vi "대회용.vi"() -> ()   [LabVIEW 2015]
uses:
  <vilib>/NXT/Block Support/NXT_OutputPort.ctl
  <vilib>/NXT/Block Support/NXT_InputPort.ctl
  <vilib>/NXT/Dual Mode Library/Sensors/EV3_Ultrasonic_CM.vi
  <vilib>/NXT/NXTIO Xnodes/NXTIONodeSubVIs/NXTMoveMotors.vi
  <vilib>/NXT/Dual Mode Library/Waits/Wait_Num.vi
  <vilib>/NXT/Dual Mode Library/Sensors/EV3_Color_Reflect.vi
  <vilib>/NXT/Subs/LVHSConnector.ctl
  <vilib>/NXT/NXTIO Xnodes/NXTIOXNode/NXTIO.xnode
  <vilib>/NXT/LegoClasses/BrickReference/BrickReference.lvclass
panel:
  in  "Power/Speed 20":i8=75
  in  "Motors 10":T1=2 items=["Port A", "Port B", "Port C", "Port D"]
  in  "Time (1 sec) 10":sgl=1.0
  in  "Power/Speed 19":i8=75
  in  "Power/Speed 18":i8=75
  in  "Motors 9":T1=2 items=["Port A", "Port B", "Port C", "Port D"]
  in  "Time (1 sec) 9":sgl=1.0
  in  "Power/Speed 17":i8=75
  in  "Power/Speed 16":i8=75
  in  "Motors 8":T1=2 items=["Port A", "Port B", "Port C", "Port D"]
  in  "Time (1 sec) 8":sgl=1.0
  in  "Power/Speed 15":i8=75
  in  "Power/Speed 14":i8=75
  in  "Motors 7":T1=2 items=["Port A", "Port B", "Port C", "Port D"]
  in  "Time (1 sec) 7":sgl=1.0
  in  "Power/Speed 13":i8=75
  in  "stop":bool
  in  "Power/Speed 1":i8=75
  in  "Motors":T1=2 items=["Port A", "Port B", "Port C", "Port D"]
  in  "Time (1 sec)":sgl=1.0
  in  "Power/Speed 6":i8=75
  in  "Power/Speed 2":i8=75
  in  "Motors 2":T1=2 items=["Port A", "Port B", "Port C", "Port D"]
  in  "Time (1 sec) 2":sgl=1.0
  in  "Power/Speed 7":i8=75
  in  "Power/Speed 3":i8=75
  in  "Motors 3":T1=2 items=["Port A", "Port B", "Port C", "Port D"]
  in  "Time (1 sec) 3":sgl=1.0
  in  "Power/Speed 8":i8=75
  in  "Power/Speed 4":i8=75
  in  "Motors 4":T1=2 items=["Port A", "Port B", "Port C", "Port D"]
  in  "Time (1 sec) 4":sgl=1.0
  in  "Power/Speed 9":i8=75
  in  "Power/Speed 5":i8=75
  in  "Motors 5":T1=2 items=["Port A", "Port B", "Port C", "Port D"]
  in  "Time (1 sec) 5":sgl=1.0
  in  "Power/Speed 10":i8=75
  in  "Power/Speed 11":i8=75
  in  "Motors 6":T1=2 items=["Port A", "Port B", "Port C", "Port D"]
  in  "Time (1 sec) 6":sgl=1.0
  in  "Power/Speed 12":i8=75
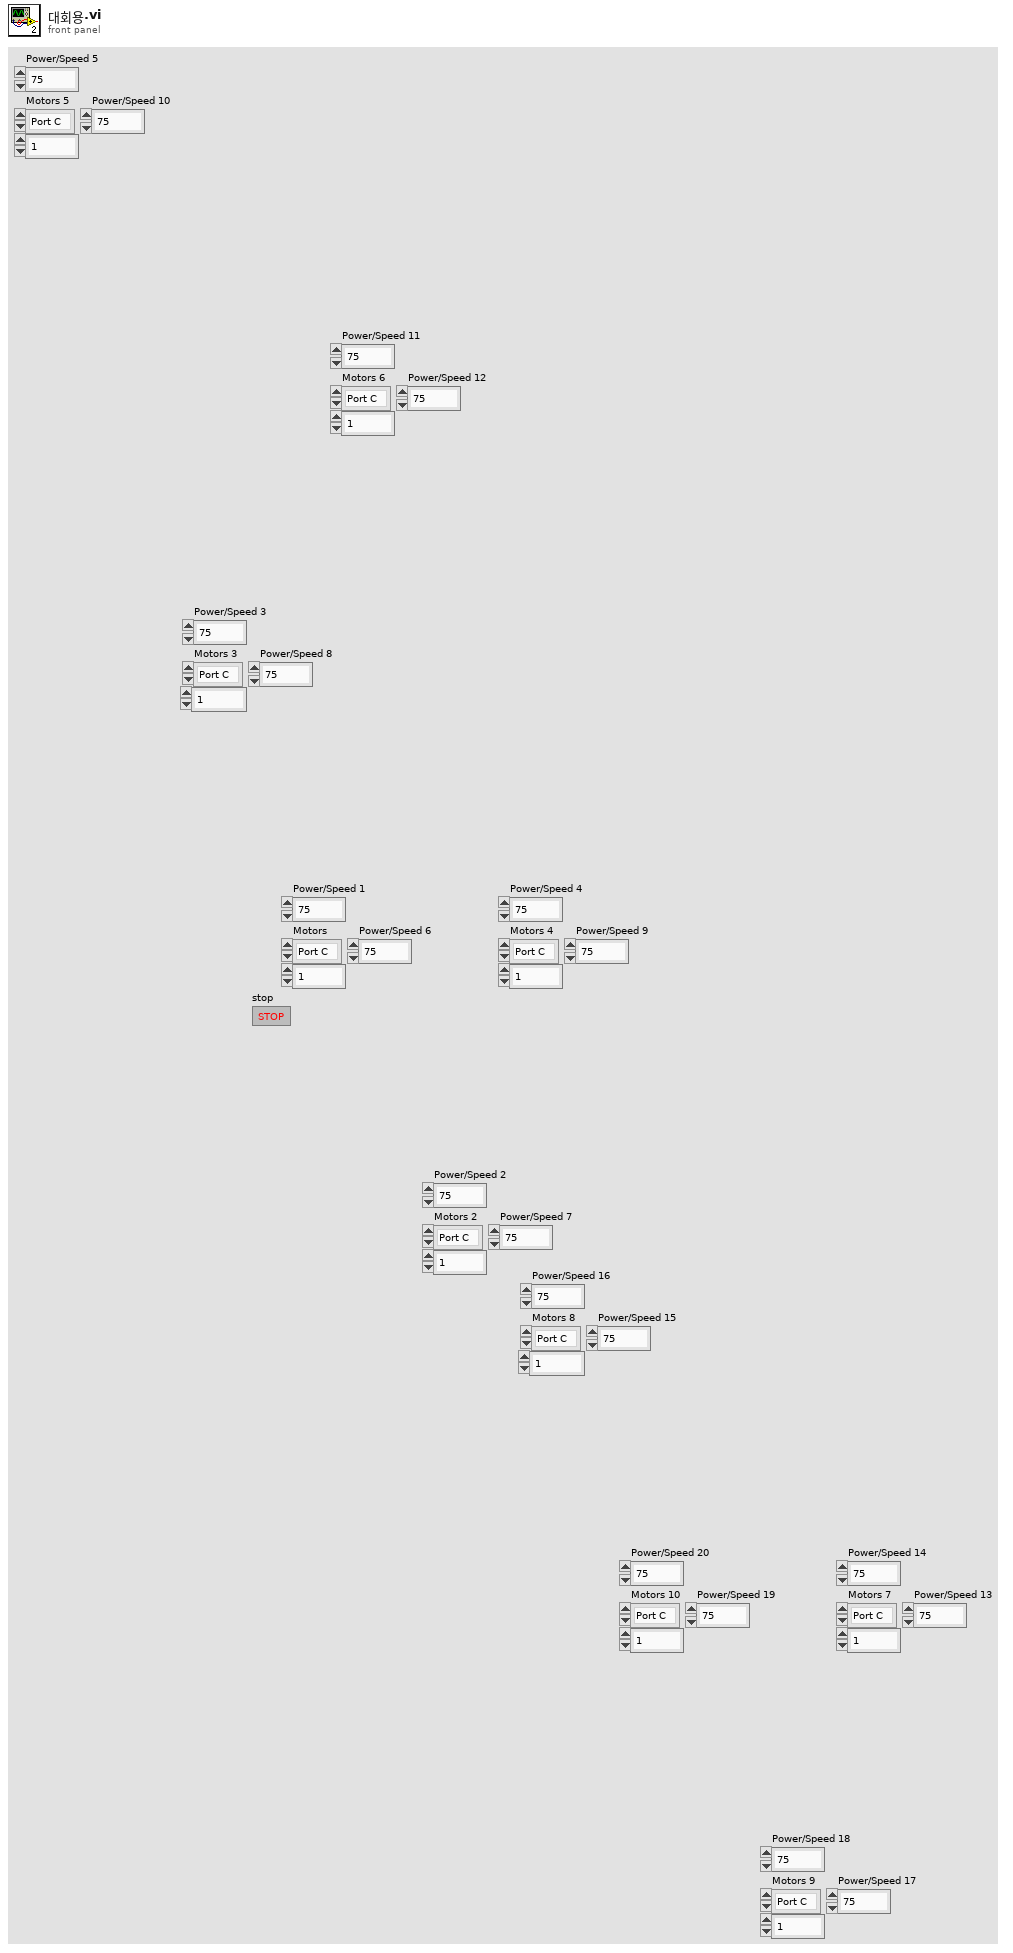
[diagram p1: front panel]
types:
  T1 = typedef "NXT_OutputPort.ctl" = u8
  T2 = typedef "NXT_InputPort.ctl" = u32
  T3 = typedef "LVHSConnector.ctl" = refnum<class "BrickReference.lvclass">
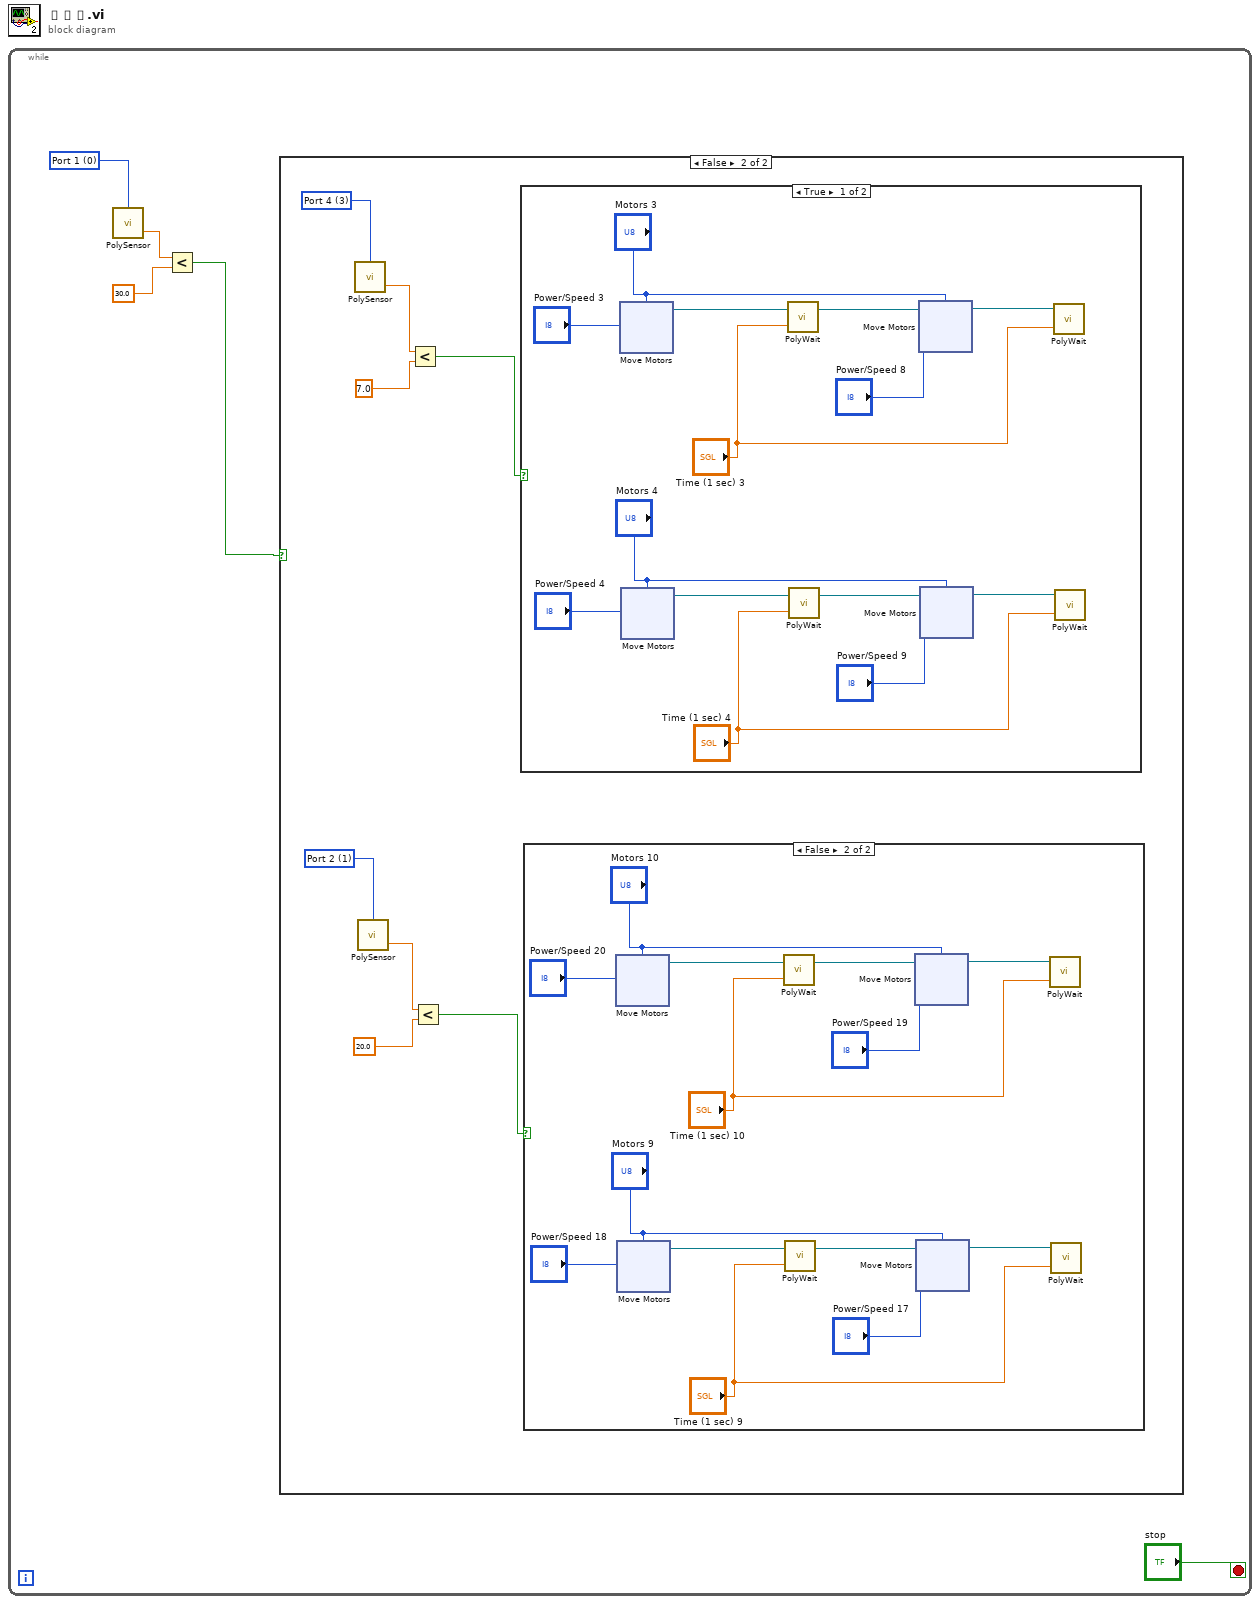
[diagram p0: block diagram]
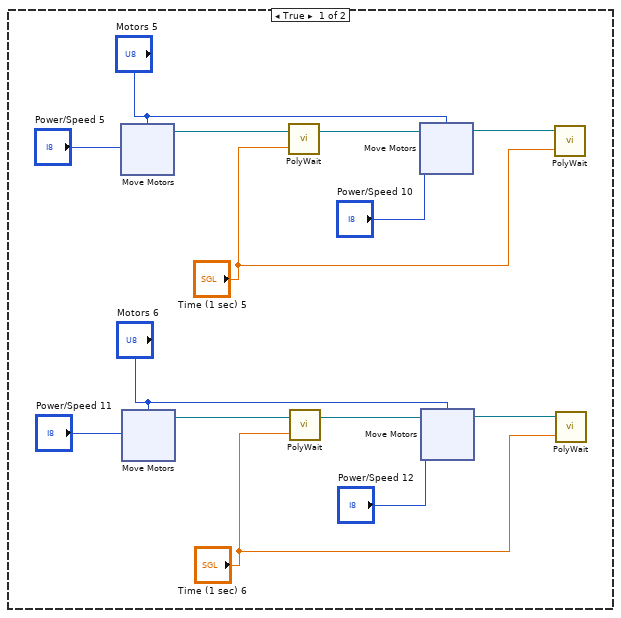
[diagram p2: hidden frame]
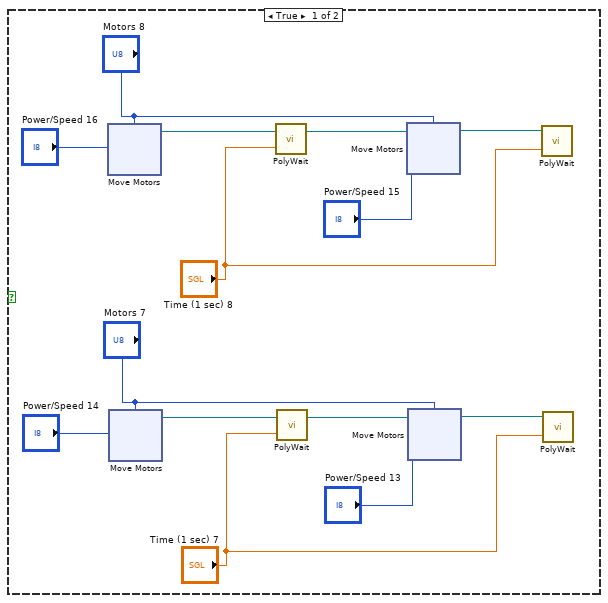
[diagram p3: hidden frame]
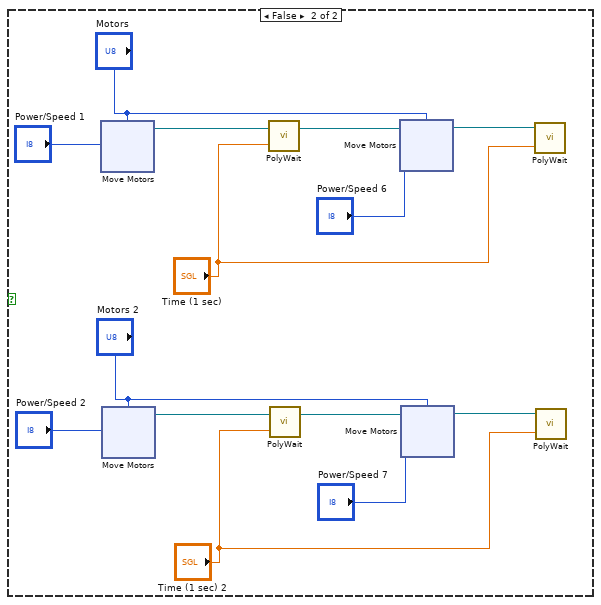
[diagram p4: hidden frame]
diagram:
  n1 = while {
    stop <- "stop" stop-if-true
    w2 = T2 0 items=["Port 1", "Port 2", "Port 3", "Port 4"] ("Port (Port 4)")
    n2 = call-poly <vilib>:"PolySensor.vi"("Port (Port 1)"=w2) -> ("Centimeters"=w4:sgl)  [unwired: 2 in, 1 out]
    n3 = Less?(x=w4, y=sgl 30.0) -> (x < y?=w1:bool)
    n4 = case shown="False" w1 {
      frame True {
        n5 = xnode "Move Motors"("Power/Speed 1"="Power/Speed 5", "Motors"="Motors 5") -> ("NXT/EV3"=w7:T3)  [unwired: 1 in]
        n6 = xnode "Move Motors"("Power/Speed 1"="Power/Speed 11", "Motors"="Motors 6") -> ("NXT/EV3"=w14:T3)  [unwired: 1 in]
        n7 = call-poly <vilib>:"PolyWait.vi"("Time (1 sec)"="Time (1 sec) 5", "NXT/EV3"=w7) -> ("NXT/EV3"=w11:T3)  [unwired: 2 in]
        n8 = call-poly <vilib>:"PolyWait.vi"("Time (1 sec)"="Time (1 sec) 6", "NXT/EV3"=w14) -> ("NXT/EV3"=w18:T3)  [unwired: 2 in]
        n9 = xnode "Move Motors"("Power/Speed 1"="Power/Speed 10", "Motors"="Motors 5", "NXT/EV3"=w11) -> ("NXT/EV3"=w10:T3)
        n10 = xnode "Move Motors"("Power/Speed 1"="Power/Speed 12", "Motors"="Motors 6", "NXT/EV3"=w18) -> ("NXT/EV3"=w17:T3)
        n11 = call-poly <vilib>:"PolyWait.vi"("Time (1 sec)"="Time (1 sec) 5", "NXT/EV3"=w10) -> ()  [unwired: 2 in, 1 out]
        n12 = call-poly <vilib>:"PolyWait.vi"("Time (1 sec)"="Time (1 sec) 6", "NXT/EV3"=w17) -> ()  [unwired: 2 in, 1 out]
      }
      frame False {
        w51 = T2 1 items=["Port 1", "Port 2", "Port 3", "Port 4"] ("Port (Port 4)")
        w55 = T2 3 items=["Port 1", "Port 2", "Port 3", "Port 4"] ("Port (Port 4)")
        n13 = call-poly <vilib>:"PolySensor.vi"("Port (Port 1)"=w55) -> ("Scaled Value"=w53:sgl)  [unwired: 2 in, 1 out]
        n14 = call-poly <vilib>:"PolySensor.vi"("Port (Port 1)"=w51) -> ("Scaled Value"=w49:sgl)  [unwired: 2 in, 1 out]
        n15 = Less?(x=w53, y=sgl 7.0) -> (x < y?=w52:bool)
        n16 = Less?(x=w49, y=sgl 20.0) -> (x < y?=w48:bool)
        n17 = case shown="True" w52 {
          frame True {
            n18 = xnode "Move Motors"("Power/Speed 1"="Power/Speed 3", "Motors"="Motors 3") -> ("NXT/EV3"=w152:T3)  [unwired: 1 in]
            n19 = xnode "Move Motors"("Power/Speed 1"="Power/Speed 4", "Motors"="Motors 4") -> ("NXT/EV3"=w145:T3)  [unwired: 1 in]
            n20 = call-poly <vilib>:"PolyWait.vi"("Time (1 sec)"="Time (1 sec) 3", "NXT/EV3"=w152) -> ("NXT/EV3"=w148:T3)  [unwired: 2 in]
            n21 = call-poly <vilib>:"PolyWait.vi"("Time (1 sec)"="Time (1 sec) 4", "NXT/EV3"=w145) -> ("NXT/EV3"=w141:T3)  [unwired: 2 in]
            n22 = xnode "Move Motors"("Power/Speed 1"="Power/Speed 8", "Motors"="Motors 3", "NXT/EV3"=w148) -> ("NXT/EV3"=w149:T3)
            n23 = xnode "Move Motors"("Power/Speed 1"="Power/Speed 9", "Motors"="Motors 4", "NXT/EV3"=w141) -> ("NXT/EV3"=w142:T3)
            n24 = call-poly <vilib>:"PolyWait.vi"("Time (1 sec)"="Time (1 sec) 3", "NXT/EV3"=w149) -> ()  [unwired: 2 in, 1 out]
            n25 = call-poly <vilib>:"PolyWait.vi"("Time (1 sec)"="Time (1 sec) 4", "NXT/EV3"=w142) -> ()  [unwired: 2 in, 1 out]
          }
          frame False {
            n26 = xnode "Move Motors"("Power/Speed 1"="Power/Speed 1", "Motors"="Motors") -> ("NXT/EV3"=w194:T3)  [unwired: 1 in]
            n27 = xnode "Move Motors"("Power/Speed 1"="Power/Speed 2", "Motors"="Motors 2") -> ("NXT/EV3"=w187:T3)  [unwired: 1 in]
            n28 = call-poly <vilib>:"PolyWait.vi"("Time (1 sec)"="Time (1 sec)", "NXT/EV3"=w194) -> ("NXT/EV3"=w190:T3)  [unwired: 2 in]
            n29 = call-poly <vilib>:"PolyWait.vi"("Time (1 sec)"="Time (1 sec) 2", "NXT/EV3"=w187) -> ("NXT/EV3"=w183:T3)  [unwired: 2 in]
            n30 = xnode "Move Motors"("Power/Speed 1"="Power/Speed 6", "Motors"="Motors", "NXT/EV3"=w190) -> ("NXT/EV3"=w191:T3)
            n31 = xnode "Move Motors"("Power/Speed 1"="Power/Speed 7", "Motors"="Motors 2", "NXT/EV3"=w183) -> ("NXT/EV3"=w184:T3)
            n32 = call-poly <vilib>:"PolyWait.vi"("Time (1 sec)"="Time (1 sec)", "NXT/EV3"=w191) -> ()  [unwired: 2 in, 1 out]
            n33 = call-poly <vilib>:"PolyWait.vi"("Time (1 sec)"="Time (1 sec) 2", "NXT/EV3"=w184) -> ()  [unwired: 2 in, 1 out]
          }
        }
        n34 = case shown="False" w48 {
          frame True {
            n35 = xnode "Move Motors"("Power/Speed 1"="Power/Speed 16", "Motors"="Motors 8") -> ("NXT/EV3"=w68:T3)  [unwired: 1 in]
            n36 = xnode "Move Motors"("Power/Speed 1"="Power/Speed 14", "Motors"="Motors 7") -> ("NXT/EV3"=w61:T3)  [unwired: 1 in]
            n37 = call-poly <vilib>:"PolyWait.vi"("Time (1 sec)"="Time (1 sec) 8", "NXT/EV3"=w68) -> ("NXT/EV3"=w64:T3)  [unwired: 2 in]
            n38 = call-poly <vilib>:"PolyWait.vi"("Time (1 sec)"="Time (1 sec) 7", "NXT/EV3"=w61) -> ("NXT/EV3"=w57:T3)  [unwired: 2 in]
            n39 = xnode "Move Motors"("Power/Speed 1"="Power/Speed 15", "Motors"="Motors 8", "NXT/EV3"=w64) -> ("NXT/EV3"=w65:T3)
            n40 = xnode "Move Motors"("Power/Speed 1"="Power/Speed 13", "Motors"="Motors 7", "NXT/EV3"=w57) -> ("NXT/EV3"=w58:T3)
            n41 = call-poly <vilib>:"PolyWait.vi"("Time (1 sec)"="Time (1 sec) 8", "NXT/EV3"=w65) -> ()  [unwired: 2 in, 1 out]
            n42 = call-poly <vilib>:"PolyWait.vi"("Time (1 sec)"="Time (1 sec) 7", "NXT/EV3"=w58) -> ()  [unwired: 2 in, 1 out]
          }
          frame False {
            n43 = xnode "Move Motors"("Power/Speed 1"="Power/Speed 20", "Motors"="Motors 10") -> ("NXT/EV3"=w110:T3)  [unwired: 1 in]
            n44 = xnode "Move Motors"("Power/Speed 1"="Power/Speed 18", "Motors"="Motors 9") -> ("NXT/EV3"=w103:T3)  [unwired: 1 in]
            n45 = call-poly <vilib>:"PolyWait.vi"("Time (1 sec)"="Time (1 sec) 10", "NXT/EV3"=w110) -> ("NXT/EV3"=w106:T3)  [unwired: 2 in]
            n46 = call-poly <vilib>:"PolyWait.vi"("Time (1 sec)"="Time (1 sec) 9", "NXT/EV3"=w103) -> ("NXT/EV3"=w99:T3)  [unwired: 2 in]
            n47 = xnode "Move Motors"("Power/Speed 1"="Power/Speed 19", "Motors"="Motors 10", "NXT/EV3"=w106) -> ("NXT/EV3"=w107:T3)
            n48 = xnode "Move Motors"("Power/Speed 1"="Power/Speed 17", "Motors"="Motors 9", "NXT/EV3"=w99) -> ("NXT/EV3"=w100:T3)
            n49 = call-poly <vilib>:"PolyWait.vi"("Time (1 sec)"="Time (1 sec) 10", "NXT/EV3"=w107) -> ()  [unwired: 2 in, 1 out]
            n50 = call-poly <vilib>:"PolyWait.vi"("Time (1 sec)"="Time (1 sec) 9", "NXT/EV3"=w100) -> ()  [unwired: 2 in, 1 out]
          }
        }
      }
    }
  }
